vi "仓库显示.vi"(11 "仓库":i32[][](array[numeric])) -> (3 "显示栏":string[][](array[string]))   [LabVIEW 2018]
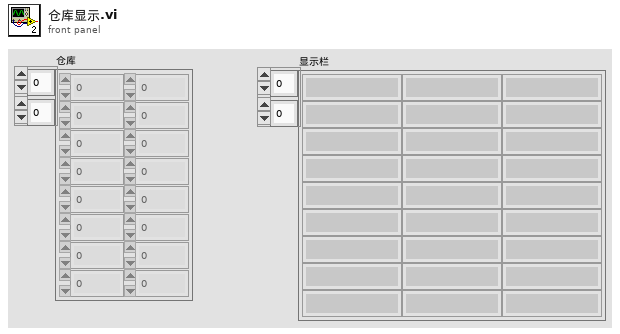
[diagram p1: front panel]
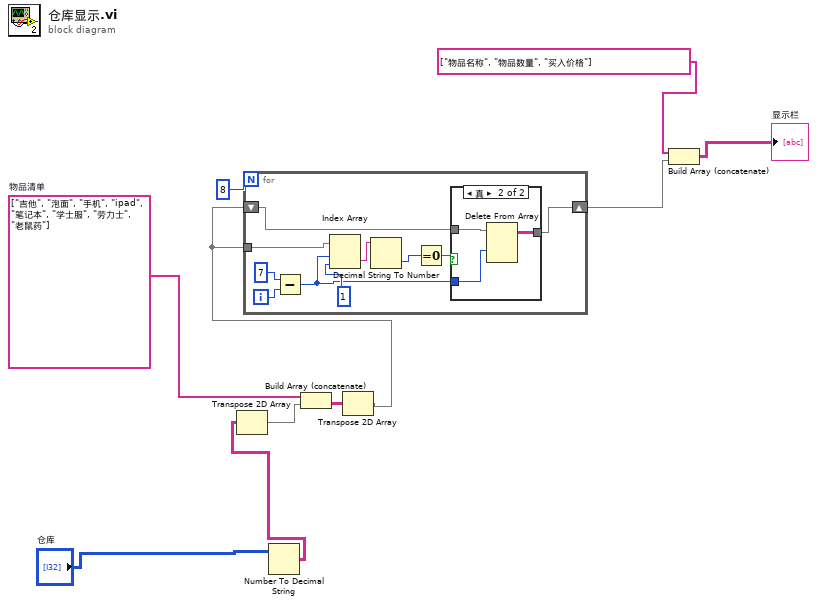
[diagram p0: block diagram]
diagram:
  w1 = string[] ["吉他", "泡面", "手机", "ipad", "笔记本", "学士服", "劳力士", "老鼠药"]  # 物品清单
  n1 = Number To Decimal String(number="仓库") -> (decimal integer string=w7:string[][])  [unwired: 1 in]
  n2 = Transpose 2D Array(2D array=w7) -> (transposed array=w6:string[][])
  n3 = Build Array (concatenate)(w1, w6) -> (w8:string[][])
  n4 = Transpose 2D Array(2D array=w8) -> (transposed array=w10:string[][])
  n5 = for {
    N: 8 -> [_]
    tunnel: w10 -> [w14]
    shift-right: [w11] -> w3
    shift-left: w10 -> [w12]
    i -> [w19]
    n6 = Subtract(x=7, y=w19) -> (x-y=w13:i32)
    n7 = Index Array(array=w14, index (row)=w13, index (col)=1) -> (element=w17:string)
    n8 = Decimal String To Number(string=w17) -> (number=w16:i32)  [unwired: 2 in, 1 out]
    n9 = Equal To 0?(x=w16) -> (x = 0?=w15:bool)
    n10 = case shown="真" w15 {
      tunnel: w12 -> [w21 w24]
      tunnel: w13 -> [_ w23]
      tunnel: [w21 w22] -> w11
      frame False {
      }
      frame True {
        n11 = Delete From Array(array=w24, index (row)=w23) -> (array with subset deleted=w22:string[][])  [unwired: 2 in, 1 out]
      }
    }
  }
  n12 = Build Array (concatenate)(string[] ["物品名称", "物品数量", "买入价格"], w3) -> (→"显示栏":string[][])
